vi "updatePanelFrame.vi"(8 "error in (no error)":errorcluster, 11 "UI in":refnum<class "UI.lvclass">) -> (0 "error out":errorcluster, 3 "UI out":refnum<class "UI.lvclass">)   [LabVIEW 2019, in "UI.lvclass"]
uses:
  UI.lvclass
  UI.lvclass/UI.ctl
  Panel/Panel.lvclass/Panel.ctl
  getPanel.vi
  getSubPanel.vi
  Panel/Panel.lvclass
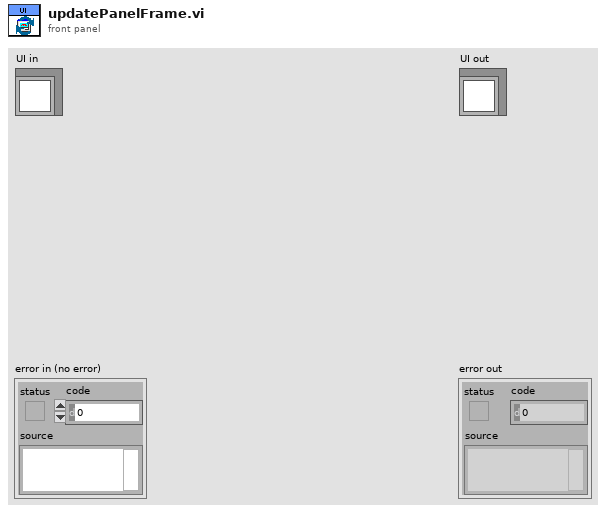
[diagram p1: front panel]
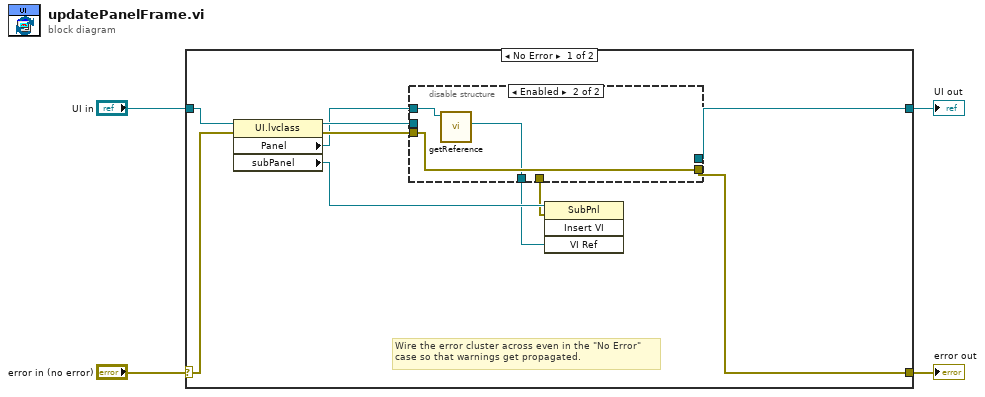
[diagram p0: block diagram]
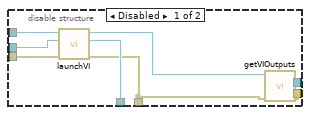
[diagram p2: hidden frame]
diagram:
  n1 = case shown="No Error" "error in (no error)" {
    selector: "error in (no error)" -> [w13 w27]
    tunnel: [w10 w27] -> w3
    tunnel: [w9 w26] -> w1
    tunnel: "UI in" -> [w14 w26]
    frame No Error {
      # "Wire the error cluster across even in the \"No Error\"\ncase so that warnings get propagated."
      n2 = property class="UI.lvclass"(reference=w14, error in=w13) -> (reference out=w12:refnum<class "UI.lvclass">, error out=w11:errorcluster, "Panel"=w7:refnum<class "Panel.lvclass">, "subPanel"=w8:refnum<vi>)
      n3 = disable-structure shown="Enabled" {
        disable-tunnel: w12 -> [w22 _]
        disable-tunnel: w11 -> [w21 w25]
        disable-tunnel: [w20 w25] -> w10
        disable-tunnel: [w19 _] -> w9
        disable-tunnel: w7 -> [w17 w24]
        disable-tunnel: [w16 w23] -> w6
        disable-tunnel: [w15 _] -> w5
        frame Disabled {
          n4 = call "launchVI.vi"("error in (no error)"=w21, "UI.lvclass"=w22, "Panel in"=w17) -> ("error out"=w15:errorcluster, "VI ref Out"=w16:refnum<vi>, "Panel out"=w18:refnum<class "Panel.lvclass">)  [unwired: 6 in]
          n5 = call "getVIOutputs.vi"("error in (no error)"=w15, "Panel in"=w18) -> ("error out"=w20:errorcluster, "UI.lvclass"=w19:refnum<class "UI.lvclass">)  [unwired: 7 in, 1 out]
        }
        frame Enabled {
          n6 = call "getReference.vi"("Panel in"=w24) -> ("Reference"=w23:refnum<vi>)  [unwired: 8 in, 2 out]
        }
      }
      n7 = invoke class="SubPnl" method="Insert VI"(reference=w8, error in=w5, "VI Ref"=w6) -> ()  [unwired: 1 in, 4 out]
    }
    frame Error {
    }
  }
  "error out" <- w3
  "UI out" <- w1
